vi "T7_Write_UINT16_Register.vi"(0 "IP Address(:port)":string="192.168.124.53", 2 "FirstChannel":u16, 4 "UINT16 to Write":u16=1) -> (9 "WrittenAt":timestamp=timestamp(3519914743.248914 s since 1904-01-01), 10 "error out":errorcluster)   [LabVIEW 2018]
panel:
  out "Starting Address":u16=2000
  # "MB Ethernet Example Master.vi\n\nInstructions\n1.Use Kipling to find your devices IP address & modify the\n\"Remote IP Addres\"\n2. Run this VI\n3. Change value of \"UINT16 to Write\" & press \"Write Data\""
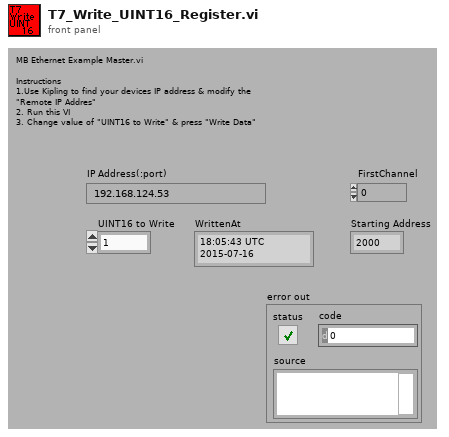
[diagram p1: front panel]
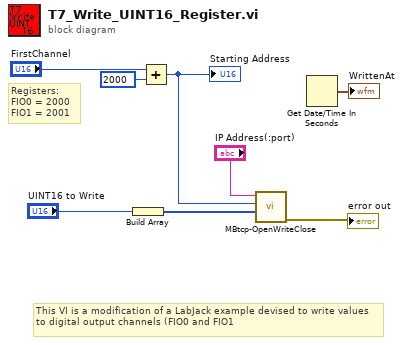
[diagram p0: block diagram]
diagram:
  # "This VI is a modification of a LabJack example devised to write values to digital output channels (FIO0 and FIO1"
  # "Registers:\nFIO0 = 2000\nFIO1 = 2001"
  n1 = Build Array("UINT16 to Write") -> (w1:u16[])
  n2 = Add(x="FirstChannel", y=u16 2000) -> (x+y=w2:u16)
  "Starting Address" <- w2
  n3 = call "MBtcp-OpenWriteClose.vi"("Values"=w1, "RegisterAddr"=w2, "IP Address(:port)"="IP Address(:port)") -> ("error out"=→"error out":errorcluster)  [unwired: 8 in]
  n4 = Get Date/Time In Seconds() -> (seconds since 1Jan1904=→"WrittenAt":timestamp)
